vi "Write To Sys Log.vi"(0 "data":variant, 7 "error in":errorcluster, 13 "format string":string) -> (4 "message":string, 8 "error out":errorcluster)   [LabVIEW 2015, in "LV System Utils v1.lvlib"]
doc: "This VI writes to the log which can be viewed by Dbgview:\nhttp://technet.microsoft.com/en-us/sysinternals/bb896647.aspx\n\nI. LOCAL DEBUGGING\n\n1. Simply start :\nDbgview.exe\n\nII. REMOTE DEBUGGING\n\n1. On the target site start:\nDbgview.exe /a /s\n\n2. On the client site start:\nDbgview.exe\n\n3. Go to Menu->Computer->Connect\n4. Type hostname of the target computer and click OK"
uses:
  LV System Utils v1.lvlib
  kernel32.dll
  <vilib>/Utility/error.llb/DialogType.ctl
  <userlib>/LV String Utils v1/LV String Utils v1.lvlib
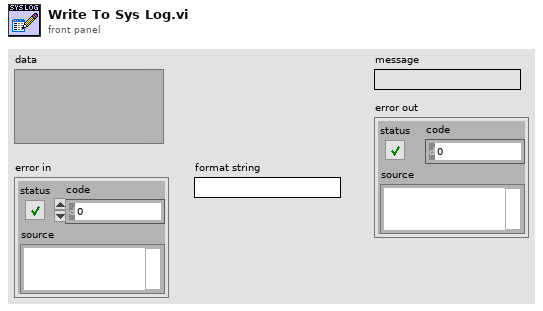
[diagram p1: front panel]
types:
  T1 = typedef "DialogType.ctl" = u16
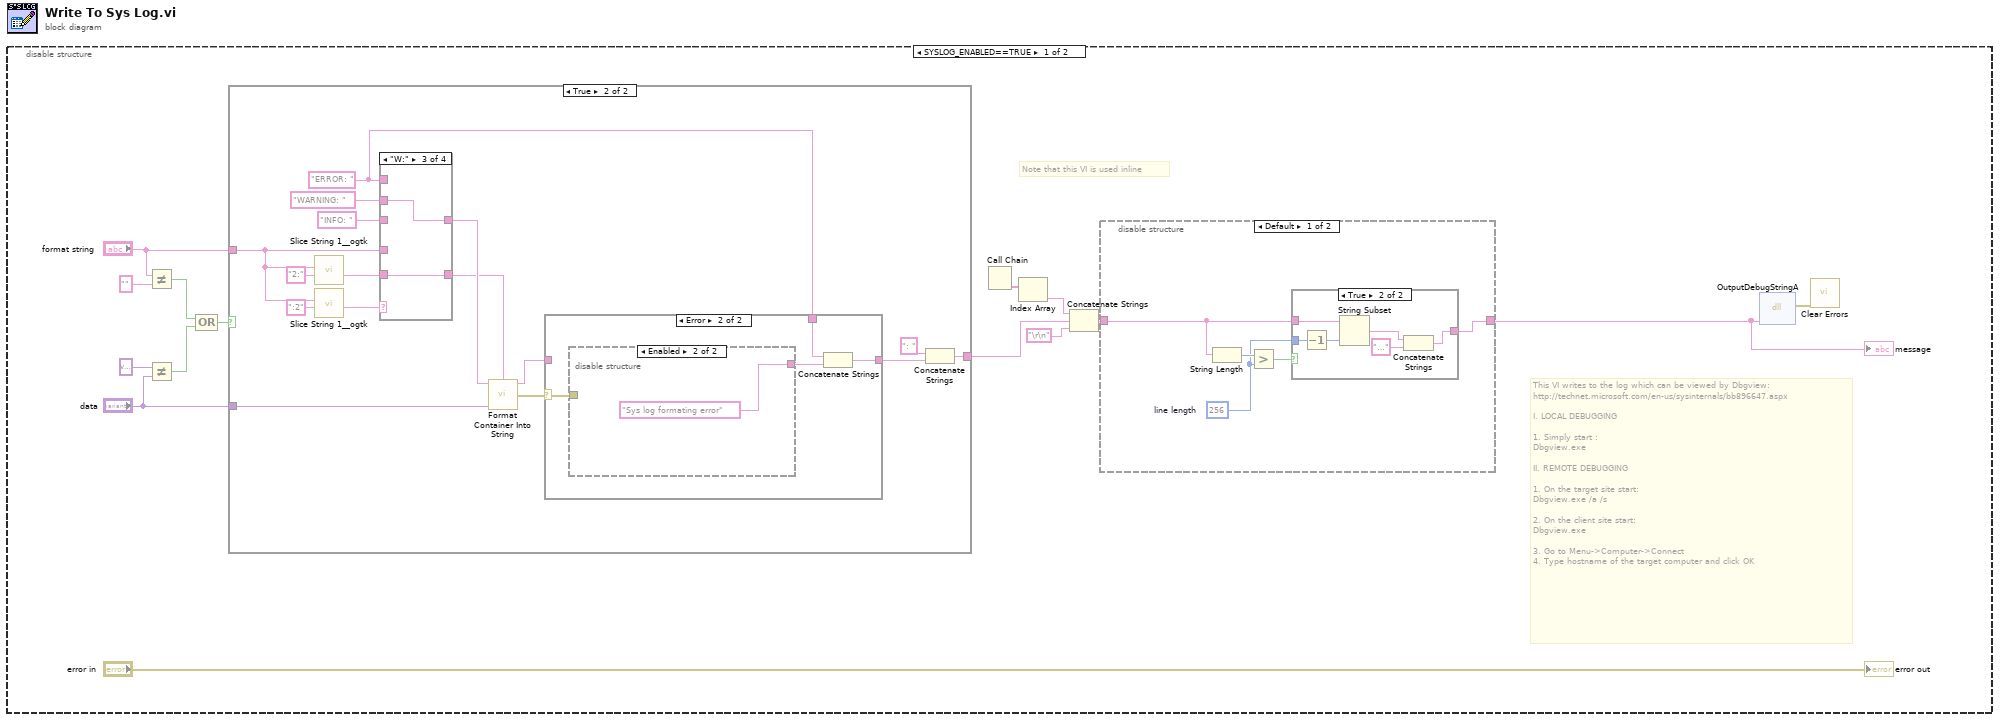
[diagram p0: block diagram]
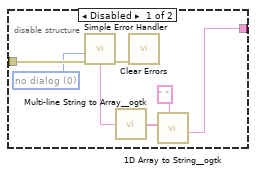
[diagram p4: hidden frame]
diagram:
  n1 = disable-structure shown="SYSLOG_ENABLED==TRUE" {
    frame condition #0 {
      # "Note that this VI is used inline"
      # "This VI writes to the log which can be viewed by Dbgview:\nhttp://technet.microsoft.com/en-us/sysinternals/bb896647.aspx\n\nI. LOCAL DEBUGGING\n\n1. Simply start :\nDbgview.exe\n\nII. REMOTE DEBUGGING\n\n1. On the target site start:\nDbgview.exe /a /s\n\n2. On the client site start:\nDbgview.exe\n\n3. Go to Menu->Computer->Connect\n4. Type hostname of the target computer and click OK"
      n2 = Not Equal?(x="format string", y="" ("format string")) -> (x != y?=w2:bool)
      n3 = Not Equal?(x=variant ("data"), y="data") -> (x != y?=w3:bool)
      n4 = Compound Arithmetic op=OR(w2, w3) -> (w1:bool)
      n5 = case shown="True" w1 {
        tunnel: [_ w31] -> w12
        tunnel: "format string" -> [_ w30]
        tunnel: "data" -> [_ w16]
        frame False {
        }
        frame True {
          w21 = "ERROR: " ("string")
          n6 = call <userlib>:"Slice String 1__ogtk.vi"("Subset (i:j)"="2:", "String"=w30) -> ("Substring (String[i:j])"=w26:string)  [unwired: 7 in]
          n7 = call <userlib>:"Slice String 1__ogtk.vi"("Subset (i:j)"=":2", "String"=w30) -> ("Substring (String[i:j])"=w27:string)  [unwired: 7 in]
          n8 = case shown="\"W:\"" w27 {
            tunnel: w30 -> [w46 _ _ _]
            tunnel: w26 -> [_ w47 w49 w51]
            tunnel: [w46 w47 w49 w51] -> w19
            tunnel: [w45 w48 w50 w52] -> w20
            tunnel: "INFO: " ("string") -> [w45 _ _ w52]
            tunnel: "WARNING: " ("string") -> [_ _ w50 _]
            tunnel: w21 -> [_ w48 _ _]
            frame Default {
            }
            frame "E:" {
            }
            frame "W:" {
            }
            frame "I:" {
            }
          }
          n9 = call <userlib>:"Format Container Into String.vi"("initial string"=w20, "format string"=w19, "input"=w16) -> ("resulting string"=w18:string, "error out"=w17:errorcluster)  [unwired: 11 in]
          n10 = case shown="Error" w17 {
            selector: w17 -> [_ w36]
            tunnel: w18 -> [w32 _]
            tunnel: [w32 w34] -> w22
            tunnel: w21 -> [_ w33]
            frame No Error {
            }
            frame Error {
              n11 = disable-structure shown="Enabled" {
                disable-tunnel: w36 -> [w43 _]
                disable-tunnel: [w37 "Sys log formating error" ("delimited string")] -> w35
                frame Disabled {
                  w42 = T1 0 items=["no dialog", "OK message", "continue or stop message", "OK message + warnings", "continue/stop + warnings"] ("type of dialog (OK msg:1)")
                  n12 = call <vilib>:"Simple Error Handler.vi"("type of dialog (OK msg:1)"=w42, "error in (no error)"=w43) -> ("error out"=w41:errorcluster, "message"=w40:string)  [unwired: 3 in, 3 out]
                  n13 = call <userlib>:"Multi-line String to Array__ogtk.vi"("string"=w40) -> ("lines"=w39:string[])
                  n14 = call <vilib>:"Clear Errors.vi"("error in (no error)"=w41) -> ()  [unwired: 5 in, 2 out]
                  n15 = call <userlib>:"1D Array to String__ogtk.vi"("delimiter (Tab)"=" ", "Array of Strings"=w39) -> ("delimited string"=w37:string)  [unwired: 9 in]
                }
                frame Enabled {
                }
              }
              n16 = Concatenate Strings(w33, w35) -> (w34:string)
            }
          }
          n17 = Concatenate Strings(": " ("separator"), w22) -> (w31:string)
        }
      }
      n18 = Call Chain() -> (call chain=w11:string[])
      n19 = Index Array(array=w11) -> (element=w10:string)  [unwired: 1 in]
      n20 = Concatenate Strings(w10, w12, "\r\n") -> (w8:string)
      n21 = disable-structure shown="Default" {
        disable-tunnel: [w54 w65] -> w9
        disable-tunnel: w8 -> [w53 w65]
        frame condition #0 (active) {
          w56 = 256  # line length
          n22 = String Length(string=w53) -> (length=w57:i32)
          n23 = Greater?(x=w57, y=w56) -> (0:w55:bool)
          n24 = case shown="True" w55 {
            tunnel: w56 -> [_ w63]
            tunnel: w53 -> [w58 w60]
            tunnel: [w58 w59] -> w54
            frame False {
            }
            frame True {
              n25 = Decrement(x=w63) -> (x-1=w64:i32)
              n26 = String Subset(string=w60, length (rest)=w64) -> (substring=w61:string)  [unwired: 1 in]
              n27 = Concatenate Strings(w61, "…" ("string")) -> (w59:string)
            }
          }
        }
        frame condition #1 {
        }
      }
      "message" <- w9
      n28 = dll-call lib="Kernel32.dll" fn="OutputDebugStringA"("debugString"=w9) -> (error out=w13:errorcluster)  [unwired: 5 in, 1 out]
      n29 = call <vilib>:"Clear Errors.vi"("error in (no error)"=w13) -> ()  [unwired: 5 in, 2 out]
      "error out" <- "error in"
    }
    frame condition #1 (active) {
    }
  }
